vi "Process.vi"(8 "error in (no error)":errorcluster, 10 "Pound in":refnum<class "Pound.lvclass">, 11 "Qbus in":refnum<class "Qbus.lvclass">) -> (0 "error out":errorcluster)   [LabVIEW 2017, in "DeviceHealth.lvlib"]
doc: "This process prepares hardware system information to be published as tags that NI InsightCM Server services can read. Every thirty seconds, this process reads values from two sources and writes them to a point-value map for publishing."
uses:
  <vilib>/addons/InsightCM/Devices/Shared/Common/DeviceHealth/DeviceHealth.lvlib
  <vilib>/addons/Qbus/Qbus.lvclass
  <vilib>/NI/Software Watchdog/Pound/Pound.lvclass
  <vilib>/addons/InsightCM/Devices/Shared/Common/DeviceHealth/controls/config.ctl
  <vilib>/addons/InsightCM/Devices/Shared/Common/DeviceHealth/controls/deviceHealthTag.ctl
  <vilib>/addons/InsightCM/Devices/Shared/Common/DeviceHealth/controls/SystemHealthTagEnum.ctl
  <vilib>/addons/InsightCM/MessageBus/Base/controls/Tag.ctl
  <vilib>/addons/InsightCM/MessageBus/Base/controls/KeyValuePair.ctl
  <vilib>/addons/TimerProcess/controls/taskType.ctl
  <vilib>/addons/TraceLogger/TraceLogger.lvlib
  <vilib>/NI/Software Watchdog/Watchdog/Watchdog.lvclass
  <vilib>/addons/InsightCM/Devices/Shared/Common/FpgaBitfileManager/FpgaBitfileManager.lvlib
  <vilib>/addons/SystemInfoProcess/SystemInfoProcess.lvlib
  <vilib>/addons/InsightCM/Devices/Shared/Common/ServerComm/ServerComm.lvlib
  <vilib>/nisyscfg/nisyscfg.lvlib
  <vilib>/addons/TimerProcess/TimerProcess.lvlib
  <vilib>/addons/InsightCM/Devices/Shared/Common/Benchmarking/Benchmarking.lvlib
  <vilib>/addons/InsightCM/Utilities/GlobalConfiguration/GlobalConfiguration.lvlib
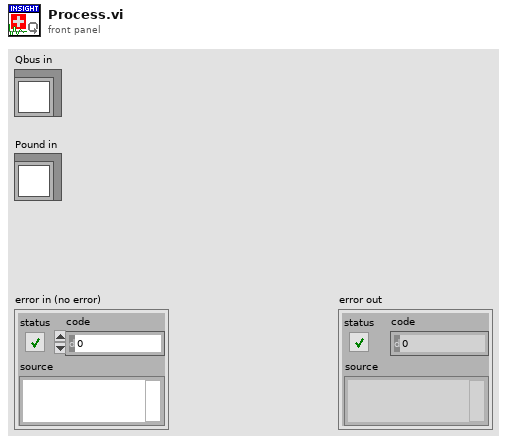
[diagram p1: front panel]
types:
  T1 = typedef "DeviceHealth.lvlib/config.ctl" = cluster{"Dynamic FPGA VI Ref":refnum<k20>, "SystemTags":T2[], "device name":string}
  T2 = typedef "DeviceHealth.lvlib/deviceHealthTag.ctl" = cluster{"SystemTags":T3, "TagId":string, "Tag":T4}
  T3 = typedef "DeviceHealth.lvlib/SystemHealthTagEnum.ctl" = enum16{"CPU Utilization", "Memory Utilization", "Disk Utilization", "Total Physical Memory", "Primary Disk Free", "Chassis Temperature", "LowRateCount"}
  T4 = typedef "Tag.ctl" = cluster{"Id":string, "Path":string, "Name":string, "Datatype":string, "Props":T5[], "Keywords":string[]}
  T5 = typedef "KeyValuePair.ctl" = cluster{"Key":string, "Value":string}
  T6 = typedef "TimerProcess.lvlib/taskType.ctl" = enum16{"single", "repeat"}
  T7 = typedef "PointValueMap.lvlib/PointMap.ctl" = refnum<data-value>
  T8 = typedef "SystemInfoProcess.lvlib/SystemResources.ctl" = cluster{"TotalPhysicalMemory":dbl, "FreePhysicalMemory":dbl, "LargestAvailableMemoryBlock":dbl, "TotalVirtualMemory":dbl, "FreeVirtualMemory":dbl, "PrimaryDiskCapacity":dbl, "PrimaryDiskFree":dbl, "Utilization":T9, "CPU Loads":T10[]}
  T9 = typedef "SystemInfoProcess.lvlib/Utilization.ctl" = cluster{"CPU":dbl, "Memory":dbl, "Disk":dbl}
  T10 = typedef "SystemInfoProcess.lvlib/CPULoad.ctl" = cluster{"Total (%)":dbl, "Time Critical (%)":dbl, "Timed Structures (%)":dbl, "High (%)":dbl, "Above Normal (%)":dbl, "Normal (%)":dbl, "Background (%)":dbl, "Idle (%)":dbl, "ISR (%)":dbl}
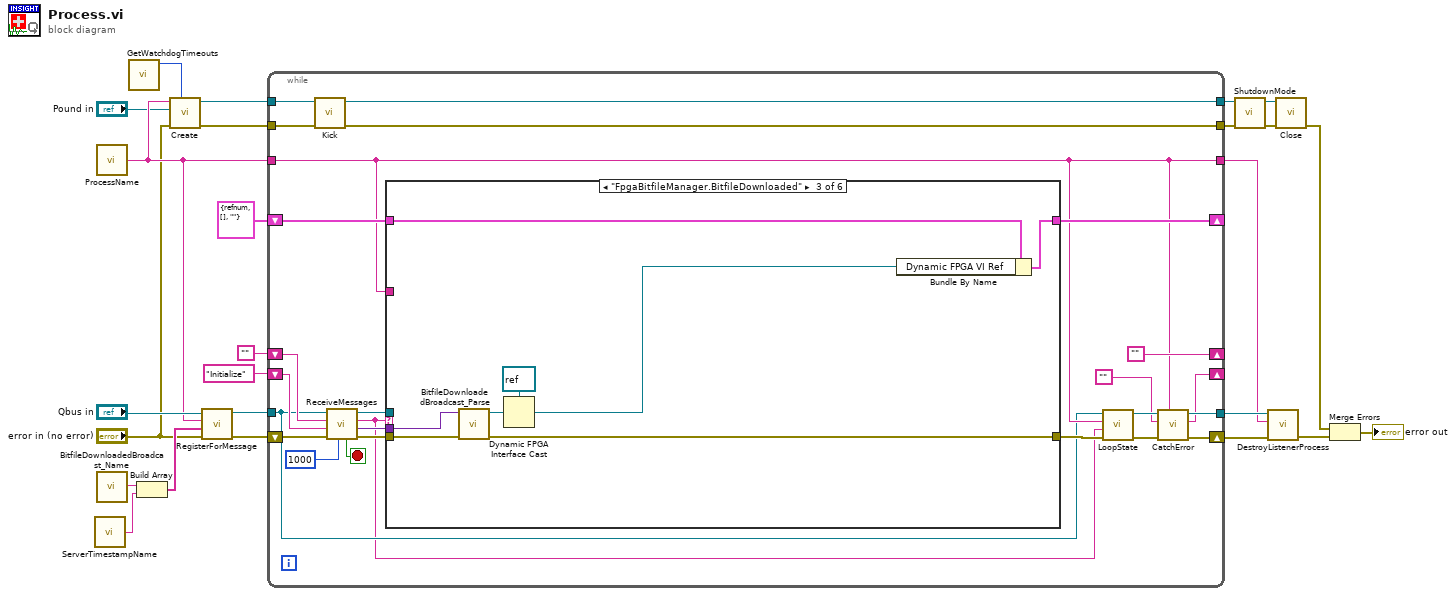
[diagram p0: block diagram]
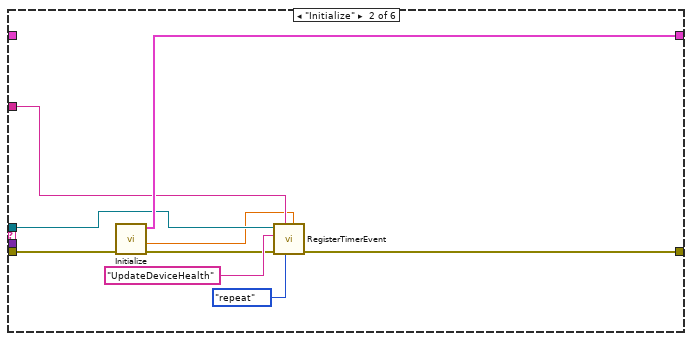
[diagram p3: hidden frame]
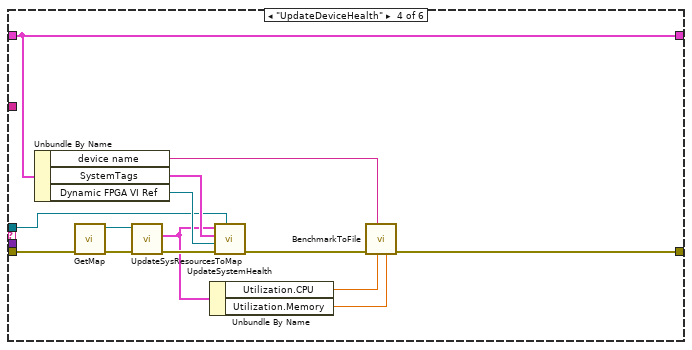
[diagram p4: hidden frame]
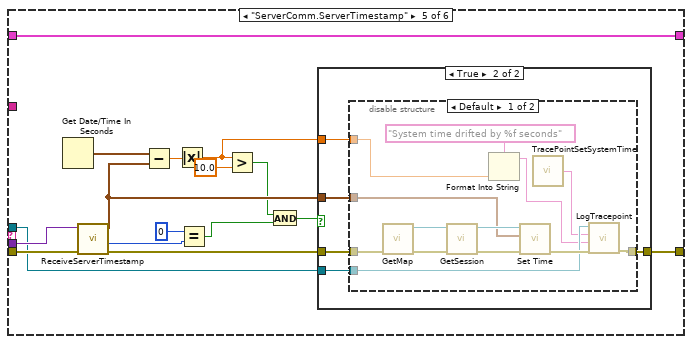
[diagram p5: hidden frame]
diagram:
  n1 = call <vilib>:"ServerTimestampName.vi"() -> ("message name"=w2:string)  [unwired: 5 in]
  n2 = call <vilib>:"ProcessName.vi"() -> ("process name"=w15:string)  [unwired: 5 in]
  n3 = call <vilib>:"BitfileDownloadedBroadcast_Name.vi"() -> ("message name"=w3:string)  [unwired: 5 in]
  n4 = call <vilib>:"GetWatchdogTimeouts.vi"() -> ("software timeout"=w1:u32)  [unwired: 10 in, 1 out]
  n5 = Build Array(w3, w2) -> (w16:string[])
  n6 = call <vilib>:"Create.vi"("Execution Timeout (ms)"=w1, "error in (no error)"="error in (no error)", "Pound"="Pound in", "Name"=w15) -> ("error out"=w9:errorcluster, "Watchdog"=w14:refnum<data-value>)  [unwired: 6 in]
  n7 = call <vilib>:"RegisterForMessage.vi"("error in (no error)"="error in (no error)", "message names"=w16, "process name"=w15, "Qbus in"="Qbus in") -> ("error in (no error)"=w24:errorcluster, "Qbus out"=w23:refnum<class "Qbus.lvclass">)  [unwired: 6 in]
  n8 = while {
    shift-right: [""] -> _
    shift-left: "" -> [w49]
    tunnel: w23 -> [w36]
    tunnel: w15 -> [w37]
    tunnel: [w40] -> w21
    tunnel: [w37] -> w20
    shift-right: [w39] -> _
    shift-left: "Initialize" -> [w44]
    shift-right: [w42] -> _
    shift-left: T1 {"Dynamic FPGA VI Ref"=refnum, "SystemTags"=[], "device name"=""} ("config") -> [w43]
    tunnel: w14 -> [w35]
    tunnel: [w34] -> w11
    tunnel: w9 -> [w33]
    tunnel: [w31] -> w8
    shift-right: [w41] -> w22
    shift-left: w24 -> [w32]
    stop <- w50 stop-if-true
    n9 = call <vilib>:"Kick.vi"("error in (no error)"=w33, "Watchdog"=w35) -> ("error out"=w31:errorcluster, "Watchdog"=w34:refnum<data-value>)  [unwired: 8 in]
    n10 = call <vilib>:"ReceiveMessages.vi"("Timeout(100)"=1000 ("milliseconds to wait"), "error in (no error)"=w32, "Priority Action"=w44, "Default Action"=w49, "Qbus in"=w36) -> ("error out"=w48:errorcluster, "MsgValue"=w45:variant, "Action"=w30:string, "Qbus out"=w46:refnum<class "Qbus.lvclass">, "Exit"=w50:bool)  [unwired: 2 in]
    n11 = case shown="\"FpgaBitfileManager.BitfileDownloaded\"" w30 {
      tunnel: w48 -> [w52 w61 w65 w79 w88 w121]
      tunnel: w46 -> [_ w57 _ w70 w85 _]
      tunnel: [w52 w53 w62 w75 w87 w121] -> w38
      tunnel: w45 -> [_ _ w64 _ w86 _]
      tunnel: w43 -> [w51 _ w63 w83 w99 w120]
      tunnel: [w51 w58 w68 w83 w99 w120] -> w42
      tunnel: w37 -> [_ w55 _ _ _ _]
      frame "", Default {
      }
      frame "Initialize" {
        n12 = call <vilib>:"Initialize.vi"("error in (no error)"=w61) -> ("error out"=w59:errorcluster, "update interval"=w54:dbl, "config"=w58:T1)  [unwired: 8 in]
        n13 = call <vilib>:"RegisterTimerEvent.vi"("interval (sec)"=w54, "type"=taskType."repeat", "process name"=w55, "error in (no error)"=w59, "callback action"="UpdateDeviceHealth", "qbus in"=w57) -> ("error out"=w53:errorcluster)  [unwired: 4 in, 1 out]
      }
      frame "FpgaBitfileManager.BitfileDownloaded" {
        n14 = call <vilib>:"BitfileDownloadedBroadcast_Parse.vi"("error in (no error)"=w65, "data"=w64) -> ("error out"=w62:errorcluster, "FPGA reference"=w66:refnum<k20>)  [unwired: 8 in]
        n15 = Dynamic FPGA Interface Cast(Session In=refnum<k20> refnum ("Dynamic FPGA VI Ref"), Type=w66) -> (Session Out=w67:refnum<k20>)
        n16 = Bundle By Name(cluster=w63, "Dynamic FPGA VI Ref"=w67) -> (w68:T1)
      }
      frame "UpdateDeviceHealth" {
        n17 = Unbundle By Name(w83) -> ("device name"=w71:string, "SystemTags"=w82:T2[], "Dynamic FPGA VI Ref"=w77:refnum<k20>)
        n18 = call <vilib>:"GetMap.vi"("error in (no error)"=w79) -> ("error out"=w81:errorcluster, "SystemInfoMap"=w78:T7)  [unwired: 9 in]
        n19 = call <vilib>:"UpdateSysResourcesToMap.vi"("error in (no error)"=w81, "map in"=w78) -> ("error out"=w80:errorcluster, "system resources"=w74:T8)  [unwired: 7 in, 1 out]
        n20 = Unbundle By Name(w74) -> ("Utilization.CPU"=w73:dbl, "Utilization.Memory"=w72:dbl)
        n21 = call <vilib>:"UpdateSystemHealth.vi"("Qbus in"=w70, "error in (no error)"=w80, "fpga reference"=w77, "system tags"=w82, "system resources"=w74) -> ("error out"=w76:errorcluster)  [unwired: 6 in]
        n22 = call <vilib>:"BenchmarkToFile.vi"("Memory"=w72, "CPU"=w73, "device name"=w71, "error in (no error)"=w76) -> ("error out"=w75:errorcluster)  [unwired: 7 in]
      }
      frame "ServerComm.ServerTimestamp" {
        n23 = Get Date/Time In Seconds() -> (seconds since 1Jan1904=w94:timestamp)
        n24 = call <vilib>:"ReceiveServerTimestamp.vi"("error in (no error)"=w88, "body"=w86) -> ("error out"=w89:errorcluster, "error code"=w90:i32, "timestamp"=w98:timestamp)  [unwired: 6 in, 1 out]
        n25 = Subtract(x=w94, y=w98) -> (x-y=w95:dbl)
        n26 = Absolute Value(x=w95) -> (abs(x)=w84:dbl)
        n27 = Equal?(x=0, y=w90) -> (x = y?=w92:bool)
        n28 = Greater?(x=w84, y=10.0) -> (0:w97:bool)
        n29 = And(x=w97, y=w92) -> (x .and. y?=w93:bool)
        n30 = case shown="True" w93 {
          tunnel: w89 -> [w100 w104]
          tunnel: [w100 w105] -> w87
          tunnel: w98 -> [_ w103]
          tunnel: w85 -> [_ w102]
          tunnel: w84 -> [_ w101]
          frame False {
          }
          frame True {
            n31 = disable-structure shown="Default" {
              disable-tunnel: [w111 w119] -> w105
              disable-tunnel: w104 -> [w116 w119]
              disable-tunnel: w103 -> [w113 _]
              disable-tunnel: w102 -> [w110 _]
              disable-tunnel: w101 -> [w106 _]
              frame condition #0 {
                n32 = call <vilib>:"GetMap.vi"("error in (no error)"=w116) -> ("error out"=w115:errorcluster, "SystemInfoMap"=w114:T7)  [unwired: 9 in]
                n33 = call <vilib>:"GetSession.vi"("error in (no error)"=w115, "map"=w114) -> ("error out"=w118:errorcluster, "session"=w117:refnum<k21>)  [unwired: 8 in]
                n34 = Format Into String(format string="System time drifted by %f seconds", w106) -> (resulting string=w107:string)  [unwired: 2 in, 1 out]
                n35 = call <vilib>:"Set Time.vi"("error in (no error)"=w118, "Time"=w113, "Session in (localhost)"=w117) -> ("error out"=w112:errorcluster)  [unwired: 5 in, 3 out]
                n36 = call <vilib>:"TracePointSetSystemTime.vi"() -> ("tracepoint name"=w108:string)  [unwired: 5 in]
                n37 = call <vilib>:"LogTracepoint.vi"("error in (no error)"=w112, "log string"=w107, "tracepoint"=w108, "qbus in"=w110) -> ("error out"=w111:errorcluster)  [unwired: 6 in, 1 out]
              }
              frame condition #1 (active) {
              }
            }
          }
        }
      }
      frame "Exit" {
      }
    }
    n38 = call <vilib>:"LoopState.vi"("error in (no error)"=w38, "loop action"=w30, "process name"=w37, "Qbus in"=w36) -> ("error out"=w28:errorcluster, "Qbus out"=w27:refnum<class "Qbus.lvclass">)  [unwired: 6 in]
    n39 = call <vilib>:"CatchError.vi"("source"=w37, "error in (no error)"=w28, "next action in"="", "Qbus in"=w27) -> ("error out"=w41:errorcluster, "next action out"=w39:string, "Qbus out"=w40:refnum<class "Qbus.lvclass">)  [unwired: 5 in]
  }
  n40 = call <vilib>:"ShutdownMode.vi"("error in (no error)"=w8, "Watchdog"=w11) -> ("error out"=w10:errorcluster, "Watchdog"=w12:refnum<data-value>)  [unwired: 8 in]
  n41 = call <vilib>:"DestroyListenerProcess.vi"("error in (no error)"=w22, "process name"=w20, "Qbus in"=w21) -> ("error in (no error)"=w7:errorcluster)  [unwired: 7 in, 1 out]
  n42 = call <vilib>:"Close.vi"("error in (no error)"=w10, "Watchdog"=w12) -> ("error out"=w6:errorcluster)  [unwired: 9 in]
  n43 = Merge Errors(w6, w7) -> (→"error out":errorcluster)
